vi "Fetch Tab Pages.vi"(5 "Max Level (10)":i32, 6 "Current Level (0)":i32, 7 "Draw Controls":T4, 8 "error in (no error)":errorcluster, 9 "Pages":refnum<vi>[](array[refnum]), 10 "Parent":string, 11 "Tab Ref in":refnum<vi>) -> (0 "error out":errorcluster, 2 "Results":T1[](array[typedef]), 3 "Tab Ref out":refnum<vi>)   [LabVIEW 2023, in "VIDoc Parsing.lvlib"]
uses:
  VIDoc Parsing.lvlib
  Settings/Parser Settings/Draw Controls Cluster.ctl
  Settings/Parser Settings/Draw Option Enum.ctl
  TypeDefs/Controls Info Cluster.ctl
  <vilib>/picture/picture.llb/imagedata.ctl
  <vilib>/Utility/miscctls.llb/LVKeyTypeDef.ctl
  65cc6c1e-4fa3-40c4-af1b-ec562817ce9d.vi
  Settings/Parser Settings/Parser Settings.lvclass
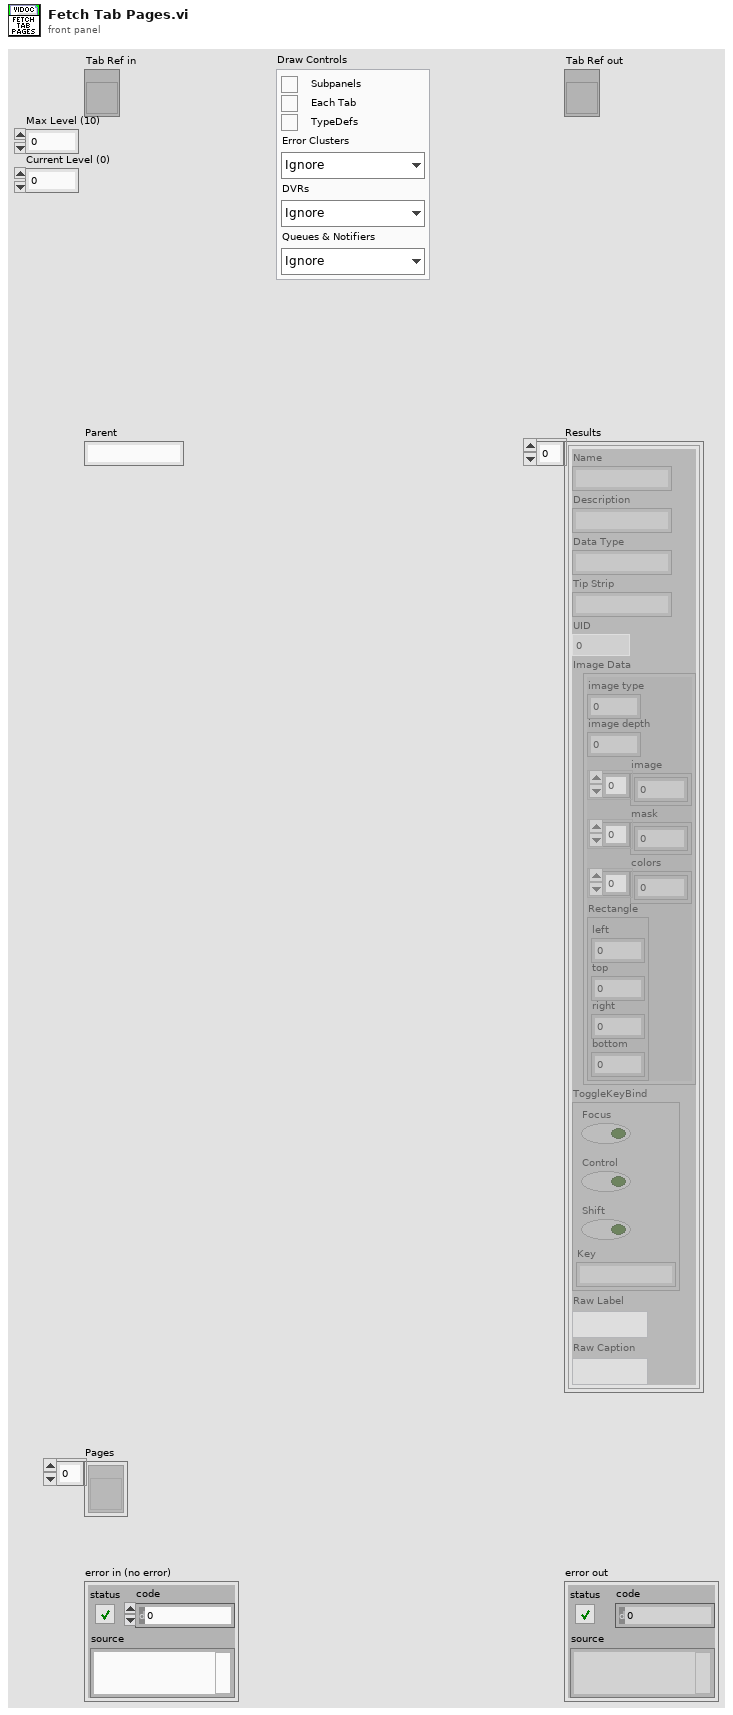
[diagram p1: front panel]
types:
  T1 = typedef "VIDoc Parsing.lvlib/Controls Info Cluster.ctl" = cluster{"Name":string, "Description":string, "Data Type":string, "Tip Strip":string, "UID":i32, "Image Data":T2, "ToggleKeyBind":T3, "Raw Label":string, "Raw Caption":string}
  T2 = typedef "imagedata.ctl" = cluster{"image type":i32, "image depth":i32, "image":u8[], "mask":u8[], "colors":u32[], "Rectangle":cluster{"left":i16, "top":i16, "right":i16, "bottom":i16}}
  T3 = typedef "LVKeyTypeDef.ctl" = cluster{"Focus":bool, "Control":bool, "Shift":bool, "Key":string}
  T4 = typedef "VIDoc Parsing.lvlib/Parser Settings.lvclass/Draw Controls Cluster.ctl" = cluster{"Subpanels":bool, "Tabs":bool, "TypeDefs":bool, "Error Clusters":T5, "DVRs":T5, "Queues & Notifiers":T5}
  T5 = typedef "VIDoc Parsing.lvlib/Parser Settings.lvclass/Draw Option Enum.ctl" = enum16{"Ignore", "Draw", "Draw + Contents"}
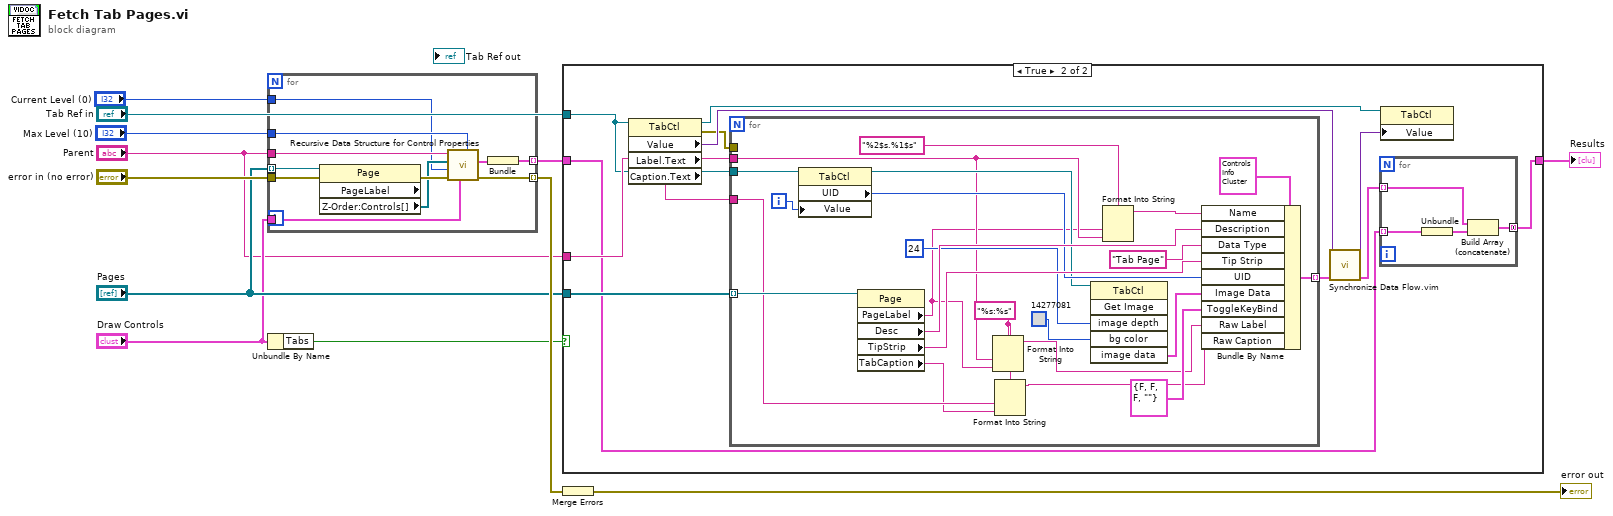
[diagram p0: block diagram]
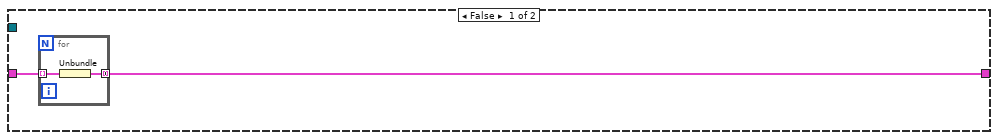
[diagram p2: hidden frame]
diagram:
  n1 = for {
    tunnel: "error in (no error)" -> [w23]
    tunnel: [w20] -> w11 mode=indexing
    tunnel: "Parent" -> [w16]
    tunnel: "Draw Controls" -> [w18]
    tunnel: "Pages" -> [w22] mode=indexing
    tunnel: [w21] -> w4 mode=indexing
    tunnel: "Max Level (10)" -> [w14]
    tunnel: "Current Level (0)" -> [w13]
    n2 = property class="Page" props=["PageLabel", "Z-Order:Controls[]"](reference=w22, error in=w23) -> (error out=w19:errorcluster, "Z-Order:Controls[]"=w17:refnum<vi>[])  [unwired: 2 out]
    n3 = call "Recursive Data Structure for Control Properties.vi"("Max Level (10)"=w14, "Draw Controls"=w18, "error in"=w19, "Current Level (0)"=w13, "Controls[]"=w17, "Parent's name"=w16) -> ("error out"=w20:errorcluster, "Results"=w15:T1[])  [unwired: 4 in]
    n4 = Bundle("Results"=w15) -> (w21:cluster{"Results":T1[]})  [unwired: 1 in]
  }
  n5 = Unbundle By Name("Draw Controls") -> ("Tabs"=w7:bool)
  n6 = case shown="True" w7 {
    tunnel: "Pages" -> [_ w39]
    tunnel: "Parent" -> [_ w38]
    tunnel: "Tab Ref in" -> [_ w37]
    tunnel: w4 -> [w25 w30]
    tunnel: [w24 w29] -> w3
    frame False {
      n7 = for {
        tunnel: w25 -> [w27] mode=indexing
        tunnel: [w26] -> w24 mode=concatenating
        n8 = Unbundle(w27) -> ("Results"=w26:T1[])
      }
    }
    frame True {
      n9 = property class="TabCtl" props=["Value", "Label", "Text", "Caption", "Text"](reference=w37) -> (reference out=w33:refnum<vi>, error out=w32:errorcluster, "Value"=w36:variant, "Caption.Text"=w28:string)  [unwired: 1 in, 1 out]
      n10 = for {
        tunnel: w39 -> [w55] mode=indexing
        tunnel: [w65] -> w34 mode=indexing
        tunnel: w38 -> [w51]
        tunnel: w37 -> [w59]
        tunnel: w32 -> [_]
        tunnel: w28 -> [w49]
        i -> [w57]
        w45 = "%s:%s" ("format string")
        n11 = property class="TabCtl"(reference=w59, "Value"=w57) -> (reference out=w54:refnum<vi>, "UID"=w58:i32)  [unwired: 1 in, 1 out]
        n12 = property class="Page"(reference=w55) -> ("PageLabel"=w50:string, "Desc"=w62:string, "TipStrip"=w60:string, "TabCaption"=w48:string)  [unwired: 1 in, 2 out]
        n13 = Format Into String(format string=w45, w51, w50) -> (resulting string=w47:string)  [unwired: 2 in, 1 out]
        n14 = Format Into String(format string=w45, w49, w48) -> (resulting string=w46:string)  [unwired: 2 in, 1 out]
        n15 = invoke class="TabCtl" method="Get Image"(reference=w54, "image depth"=24 ("Image Depth"), "bg color"=u32 14277081 ("Color Box")) -> ("image data"=w53:T2)  [unwired: 3 in, 5 out]
        n16 = Format Into String(format string="%2$s.%1$s", w50, w51) -> (resulting string=w63:string)  [unwired: 2 in, 1 out]
        n17 = Bundle By Name(cluster=T1 {"Name"="", "Description"="", "Data Type"="", "Tip Strip"="", "UID"=0, "Image Data"={"image type"=0, "image depth"=0, "image"=[], "mask"=[], "colors"=[], "Rectangle"={"left"=0, "top"=0, "right"=0, "bottom"=0}}, "ToggleKeyBind"={"Focus"=FALSE, "Control"=FALSE, "Shift"=FALSE, "Key"=""}, "Raw Label"="", "Raw Caption"=""}, "Name"=w63, "Description"=w62, "Data Type"="Tab Page", "Tip Strip"=w60, "UID"=w58, "Image Data"=w53, "ToggleKeyBind"=T3 {"Focus"=FALSE, "Control"=FALSE, "Shift"=FALSE, "Key"=""}, "Raw Label"=w47, "Raw Caption"=w46) -> (w65:T1)
      }
      n18 = call "Synchronize Data Flow.vim"("input 4"=w34, "input 1"=w36) -> ("output 4"=w31:T1[], "output 1"=w35:variant)  [unwired: 2 in, 2 out]
      n19 = for {
        tunnel: w31 -> [w42] mode=indexing
        tunnel: w30 -> [w43] mode=indexing
        tunnel: [w40] -> w29 mode=concatenating
        n20 = Unbundle(w43) -> ("Results"=w41:T1[])
        n21 = Build Array (concatenate)(w42, w41) -> (w40:T1[])
      }
      n22 = property class="TabCtl"(reference=w33, "Value"=w35) -> ()  [unwired: 1 in, 2 out]
    }
  }
  "Results" <- w3
  n23 = Merge Errors(w11) -> (→"error out":errorcluster)
